vi "New Data Incorporation Method Dialog.vi"() -> (2 "Always? out":bool, 3 "New Data Behavior out":T1)   [LabVIEW 2012]
doc: "Prompts the user to select which analysis routines to run and whether or not to remember the selection."
uses:
  controls/New Data Behavior.ctl
panel:
  in  "New Data Behavior":u16(ring) items=["Prompt", "Replace", "Overlay", "Append"]
  in  "OK Button":bool
  in  "Always?":bool
  # "What would you like to do with the new data?"
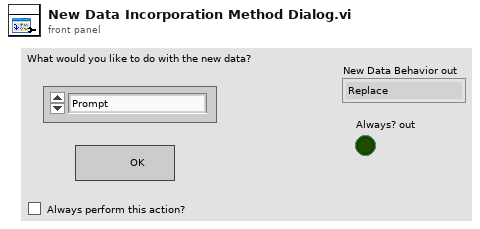
[diagram p1: front panel]
types:
  T1 = typedef "New Data Behavior.ctl" = enum16{"Replace", "Overlay", "Append"}
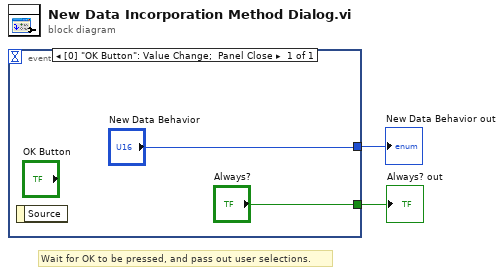
[diagram p0: block diagram]
diagram:
  # "Wait for OK to be pressed, and pass out user selections."
  n1 = event shown="[0] \"OK Button\": Value Change;  Panel Close" {
    selector: _ -> [_]
    dyn-events: _ -> [_]
    timeout: _ -> [_]
    tunnel: ["Always?"] -> w2
    tunnel: ["New Data Behavior"] -> w1
    event "OK Button": Value Change; Panel Close {
      n2 = event-data() -> ()  [unwired: 1 in, 1 out]
    }
  }
  "New Data Behavior out" <- w1
  "Always? out" <- w2
